vi "MCListbox Editor.vi"(5 "Remove Row":bool, 6 "new element/subarray":string[](array[string]), 7 "Add Row Above":bool=TRUE, 8 "Error In":errorcluster, 9 "CellBG New Cells":u32(colorbox)=16777215, 10 "CellBG Unused Cells":u32(colorbox)=16777238, 11 "MulticolumnListbox in":refnum<vi>) -> (0 "Error Out":errorcluster, 1 "Value":i32, 3 "MulticolumnListbox out":refnum<vi>)   [LabVIEW 2013]
uses:
  <vilib>/Utility/miscctls.llb/LVRowAndColumnTypeDef.ctl
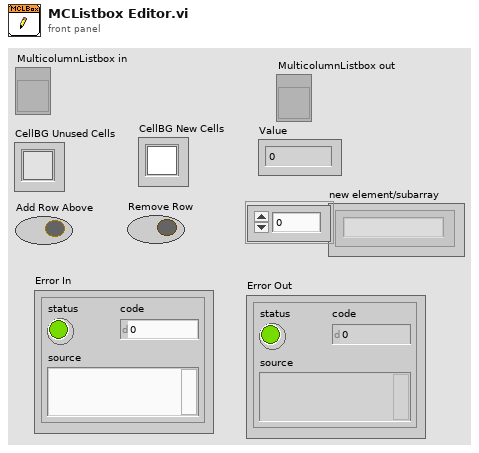
[diagram p1: front panel]
types:
  T1 = typedef "LVRowAndColumnTypeDef.ctl" = cluster{"Row":i32, "Column":i32}
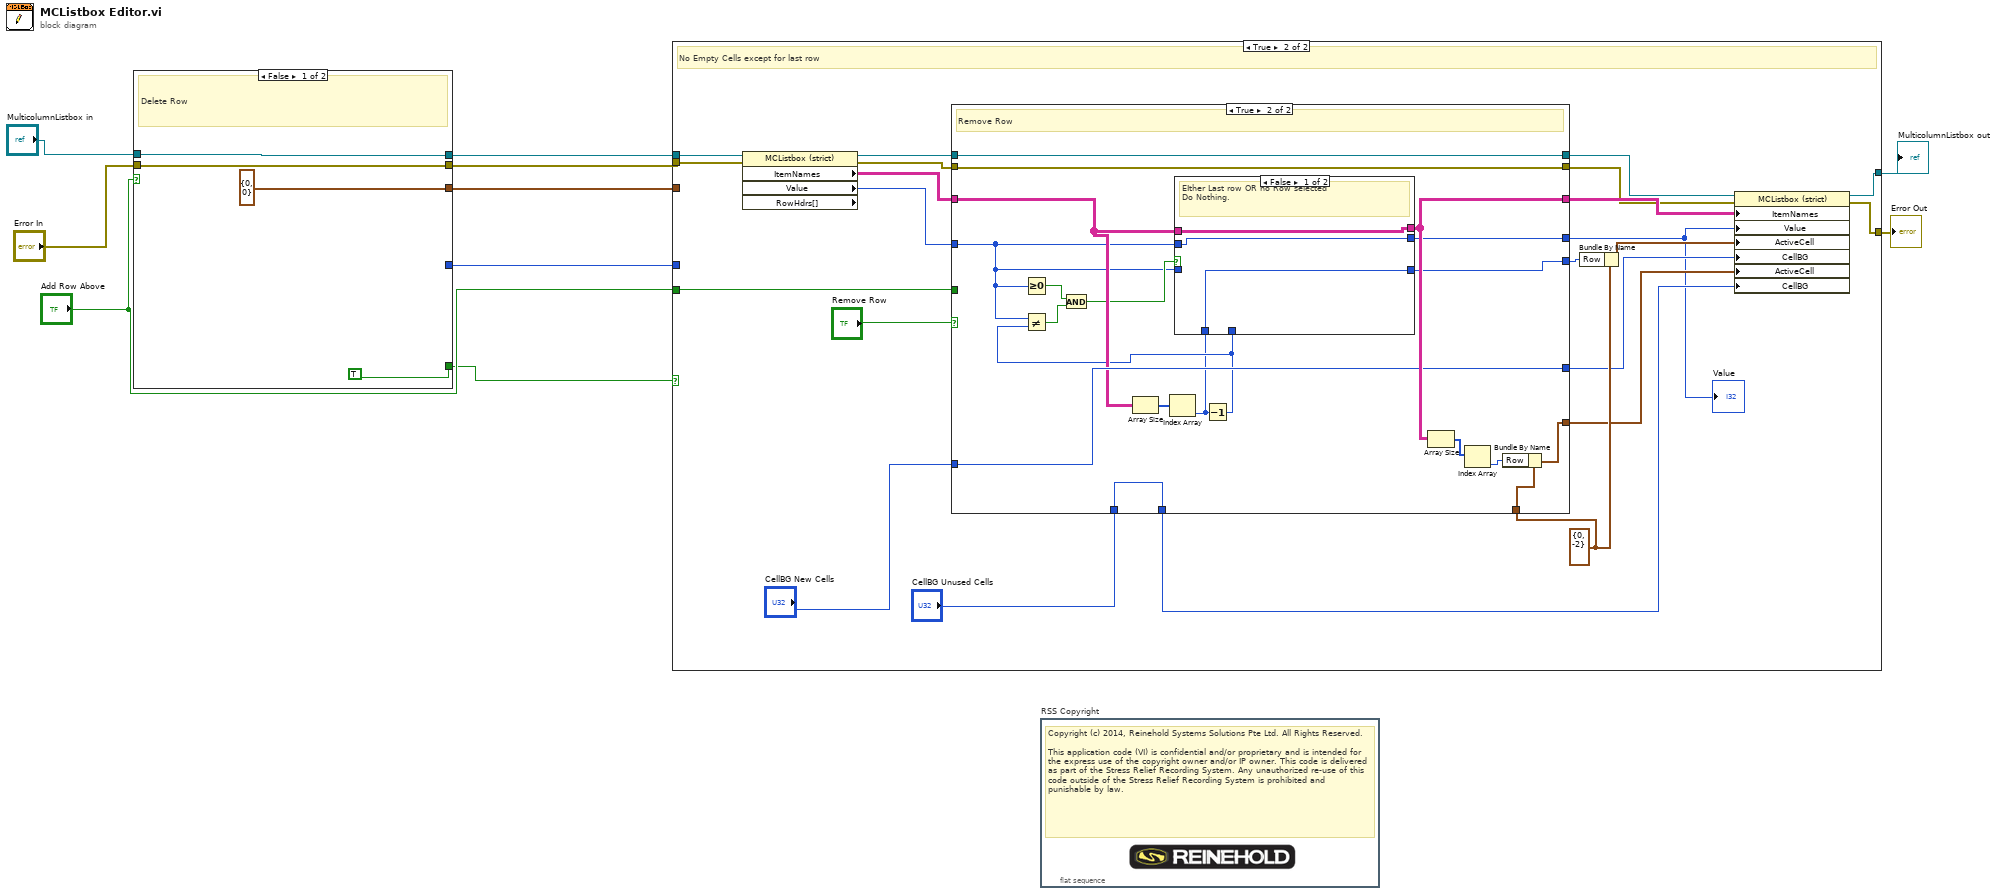
[diagram p0: block diagram]
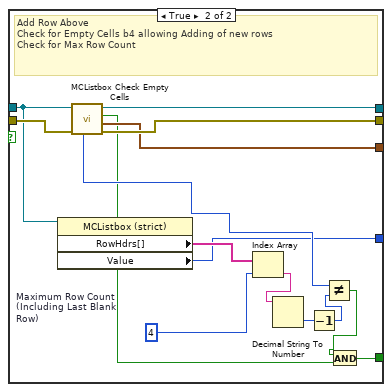
[diagram p2: hidden frame]
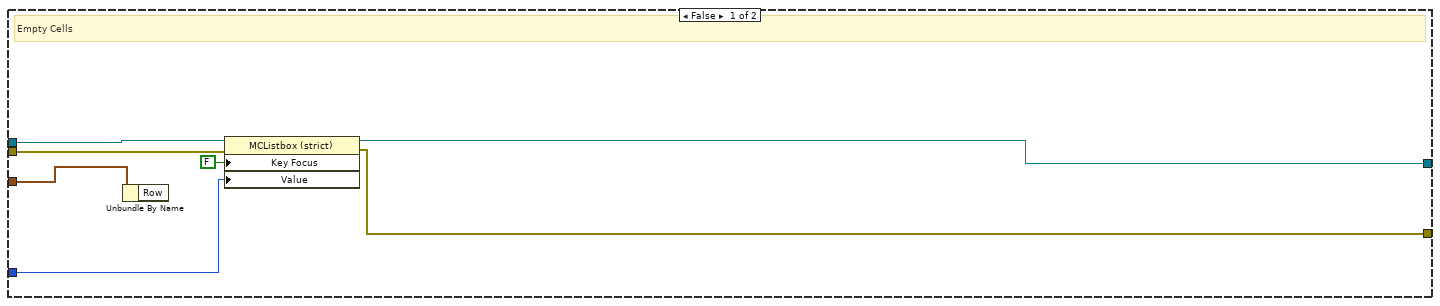
[diagram p3: hidden frame]
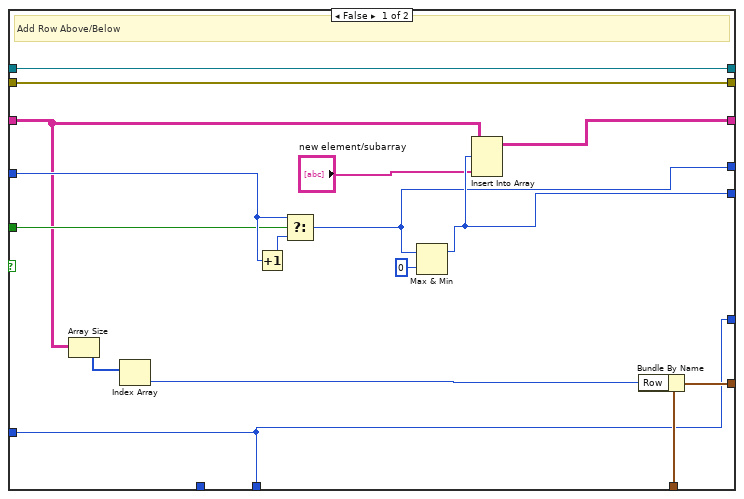
[diagram p4: hidden frame]
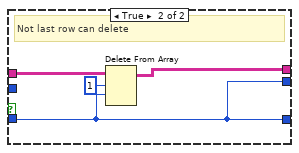
[diagram p5: hidden frame]
diagram:
  n1 = case shown="False" "Add Row Above" {
    tunnel: "MulticolumnListbox in" -> [w14 w20]
    tunnel: "Error In" -> [w13 w29]
    tunnel: [w14 w28] -> w3
    tunnel: [w13 w27] -> w7
    tunnel: [TRUE ("No Empty Cells (except for last row)") w16] -> w4
    tunnel: [T1 {"Row"=0, "Column"=0} ("Edit Position Now") w26] -> w6
    tunnel: [_ w15] -> w1
    frame False {
      # "Delete Row"
    }
    frame True {
      w22 = 4  # Maximum Row Count (Including Last Blank Row)
      # "Add Row Above\nCheck for Empty Cells b4 allowing Adding of new rows\nCheck for Max Row Count"
      n2 = property on="Property Node" class="MCListbox (strict)"(reference=w20) -> ("RowHdrs[]"=w23:string[], "Value"=w15:i32)  [unwired: 1 in, 2 out]
      n3 = call "MCListbox Check Empty Cells.vi"("Error In"=w29, "MulticolumnListbox in"=w20) -> ("Error Out"=w27:errorcluster, "Edit Position Now"=w26:T1, "No Empty Cells (except for last row)"=w17:bool, "MulticolumnListbox out"=w28:refnum<vi>, "last row"=w19:i32)  [unwired: 4 in, 1 out]
      n4 = Index Array(array=w23, index=w22) -> (element=w21:string)
      n5 = Decimal String To Number(string=w21) -> (number=w24:i32)  [unwired: 2 in, 1 out]
      n6 = Decrement(x=w24) -> (x-1=w25:i32)
      n7 = Not Equal?(x=w19, y=w25) -> (x != y?=w18:bool)
      n8 = And(x=w18, y=w17) -> (x .and. y?=w16:bool)
    }
  }
  n9 = case shown="True" w4 {
    tunnel: "Add Row Above" -> [_ w55]
    tunnel: w3 -> [w36 w52]
    tunnel: w7 -> [w35 w51]
    tunnel: [w34 w50] -> w10
    tunnel: [w33 w46] -> w9
    tunnel: w6 -> [w31 _]
    tunnel: w1 -> [w30 _]
    frame False {
      # "Empty Cells"
      n10 = Unbundle By Name(w31) -> ()  [unwired: 1 out]
      n11 = property on="Property Node" class="MCListbox (strict)"(reference=w36, error in=w35, "Key Focus"=FALSE, "Value"=w30) -> (reference out=w33:refnum<vi>, error out=w34:errorcluster)
    }
    frame True {
      w45 = T1 {"Row"=0, "Column"=-2} ("Active Cell:Active Cell")
      # "No Empty Cells except for last row"
      n12 = property on="Property Node" class="MCListbox (strict)" props=["ItemNames", "Value", "RowHdrs[]"](reference=w52, error in=w51) -> (reference out=w41:refnum<vi>, error out=w38:errorcluster, "ItemNames"=w53:string[][], "Value"=w56:i32)  [unwired: 1 out]
      n13 = case shown="True" "Remove Row" {
        tunnel: [w71 w84] -> w57
        tunnel: w56 -> [w74 w76]
        tunnel: w55 -> [w69 _]
        tunnel: [w63 w89] -> w54
        tunnel: w53 -> [w65 w83]
        tunnel: "CellBG New Cells" -> [w64 w88]
        tunnel: [w64 w93] -> w43
        tunnel: "CellBG Unused Cells" -> [_ w93]
        tunnel: w45 -> [w67 w91]
        tunnel: [w66 w90] -> w44
        tunnel: [w64 w88] -> w42
        tunnel: w41 -> [w62 w86]
        tunnel: [w62 w86] -> w40
        tunnel: [w61 w85] -> w39
        tunnel: w38 -> [w61 w85]
        tunnel: [w60 w78] -> w37
        frame False {
          # "Add Row Above/Below"
          n14 = Array Size(array=w65) -> (size(s)=w70:i32[])
          n15 = Index Array(array=w70) -> (element=w68:i32)  [unwired: 1 in]
          n16 = Increment(x=w74) -> (x+1=w73:i32)
          n17 = Select(t=w74, s=w69, f=w73) -> (s? t:f=w60:i32)
          n18 = Max & Min(x=w60, y=0) -> (max(x,y)=w71:i32)  [unwired: 1 out]
          n19 = Insert Into Array(array=w65, index (row)=w71, new element="new element/subarray") -> (w63:string[][])  [unwired: 1 in]
          n20 = Bundle By Name(cluster=w67, "Row"=w68) -> (w66:T1)
        }
        frame True {
          # "Remove Row"
          n21 = Greater Or Equal To 0?(x=w76) -> (x >= 0?=w81:bool)
          n22 = Array Size(array=w83) -> (size(s)=w82:i32[])
          n23 = Index Array(array=w82) -> (element=w75:i32)  [unwired: 1 in]
          n24 = Decrement(x=w75) -> (x-1=w77:i32)
          n25 = Not Equal?(x=w76, y=w77) -> (x != y?=w80:bool)
          n26 = Compound Arithmetic op=AND(w81, w80) -> (w79:bool)
          n27 = case shown="False" w79 {
            tunnel: [w96 w100] -> w89
            tunnel: [w95 w97] -> w84
            tunnel: w76 -> [_ w97]
            tunnel: w83 -> [w96 w98]
            tunnel: [w94 w97] -> w78
            tunnel: w77 -> [_ _]
            tunnel: w75 -> [w95 _]
            tunnel: w76 -> [w94 _]
            frame False {
              # "EIther Last row OR no Row selected\nDo Nothing."
            }
            frame True {
              # "Not last row can delete"
              n28 = Delete From Array(array=w98, length=1, index (row)=w97) -> (array with subset deleted=w100:string[][])  [unwired: 1 in, 1 out]
            }
          }
          n29 = Array Size(array=w89) -> (size(s)=w92:i32[])
          n30 = Index Array(array=w92) -> (element=w87:i32)  [unwired: 1 in]
          n31 = Bundle By Name(cluster=w91, "Row"=w87) -> (w90:T1)
        }
      }
      "Value" <- w37
      n32 = Bundle By Name(cluster=w45, "Row"=w57) -> (w58:T1)
      n33 = property on="Property Node" class="MCListbox (strict)"(reference=w40, error in=w39, "ItemNames"=w54, "Value"=w37, "ActiveCell"=w58, "CellBG"=w42, "ActiveCell"=w44, "CellBG"=w43) -> (reference out=w46:refnum<vi>, error out=w50:errorcluster)
    }
  }
  "Error Out" <- w10
  "MulticolumnListbox out" <- w9
  n34 = flat-sequence "RSS Copyright" {
    frame #0 {
      # "Copyright (c) 2014, Reinehold Systems Solutions Pte Ltd. All Rights Reserved.\n\nThis application code (VI) is confidential and/or proprietary and is intended for the express use of the copyright owner and/or IP owner. This code is delivered as part of the Stress Relief Recording System. Any unauthorized re-use of this code outside of the Stress Relief Recording System is prohibited and punishable by law."
    }
  }
